vi "SYSID_FPGA2.vi"() -> ()   [LabVIEW 2014, in "SYSID.lvlib"]
doc: "This VI was generated automatically using the FPGA Wizard. You can modify the VI normally."
uses:
  SYSID.lvlib
  <vilib>/Platform/TimedLoop/XDataNode/timing_clust.ctl
  <vilib>/Platform/TimedLoop/XDataNode/nitl_modes.ctl
  <vilib>/Platform/TimedLoop/XDataNode/wakeup.ctl
  <vilib>/rvi/FXPMathLib/FxpConvert/subVIs/nifxpmath_Convert_SimConfig.ctl
  <vilib>/fxp/LVFixedPointQuantizationPolicyTypeDef.ctl
  <vilib>/fxp/LVFixedPointOverflowPolicyTypeDef.ctl
  <vilib>/rvi/Emulation/niFpgaGetClockAttributes.vi
  <vilib>/rvi/Emulation/niFpgaSctlEmulationGetInTimedLoop.vi
  <vilib>/rvi/Emulation/niFpgaEmulationReportErrorSimple.vi
  <vilib>/rvi/Emulation/niFpgaCriticalErrorInLSC.vi
  <vilib>/rvi/Emulation/niFpgaProcessEmulError.vi
  <vilib>/rvi/eio/common/nirviEmuTemplateMethod_errors.vi
  <vilib>/rvi/FXPMathLib/FxpConvert/simVIs/DllFxpConvertTemp_sub.vi
  <vilib>/Platform/TimedLoop/XDataNode/XDataNode.xnode
  <vilib>/eio/EIONode/EIONode.xnode
  <vilib>/rvi/FXPMathLib/FxpSub/XNode/nifxpmath_Sub.xnode
  <vilib>/rvi/FXPMathLib/FxpMul/XNode/nifxpmath_Multiplier.xnode
  <vilib>/rvi/FXPMathLib/FxpAdd/XNode/nifxpmath_Add.xnode
  <vilib>/rvi/FXPMathLib/FxpConvert/XNode/nifxpmath_Convert.xnode
  <vilib>/Platform/TimedLoop/XDataNode/XDNodeRunTimeDep.lvlib
  <vilib>/rvi/FXPMathLib/sim/FxpSim.dll
panel:
  in  "State_Control":fxp<+/-,20,5>
  in  "K4":fxp<+/-,32,7>
  in  "K3":fxp<+/-,32,7>
  in  "K2":fxp<+/-,32,7>
  in  "K1":fxp<+/-,32,7>
  out "Delta_theta":fxp<+/-,33,33>
  out "Delta_X":fxp<+/-,33,33>
  out "Pendulum Position":i32
  out "_Pendulum Position":i32
  in  "Pendulum Reset":bool
  out "Amp Cpmmand":fxp<+/-,20,5>
  in  "Reference":i32
  out "Right Limit":bool
  out "Left Limit":bool
  in  "Brake":bool=TRUE
  in  "Amp Reset":bool=TRUE
  in  "Amp Enable":bool
  in  "DGain":fxp<+/-,32,7>
  in  "PGain":fxp<+/-,32,7>
  out "Error-dot":fxp<+/-,55,34>
  out "Error":fxp<+/-,33,33>
  out "Control Late? (Latched)":bool
  out "Actual Control Rate (Ticks)":u32
  in  "Control Reset":bool
  in  "Control Rate (ticks)":u32=1000 caption="Control Rate (Ticks)"
  out "quad saved (Port0/DIO0,Port0/DIO1)":cluster{"Position":i32, "Index Count":u16}
  out "Stage Position":i32
  out "_quad pos (Port0/DIO0,Port0/DIO1)":i32
  in  "quad reset (Port0/DIO0,Port0/DIO1)":bool
  out "_quad saved (Port0/DIO0,Port0/DIO1)":cluster{"Position":i32, "Index Count":u16}
  in  "AO (ModB/AO2)":fxp<+/-,20,5>
  in  "Drive Command":fxp<+/-,20,5>
  out "AI (ModA/AI0)":fxp<+/-,26,5> format="%.6g"
  in  "Local Stop 0":bool
  out "Actual Loop Rate (Ticks)":u32
  out "Late? Latched":bool
  in  "Loop Rate (Ticks)":u32=571
  in  "Reset":bool
  in  "Start 0":bool
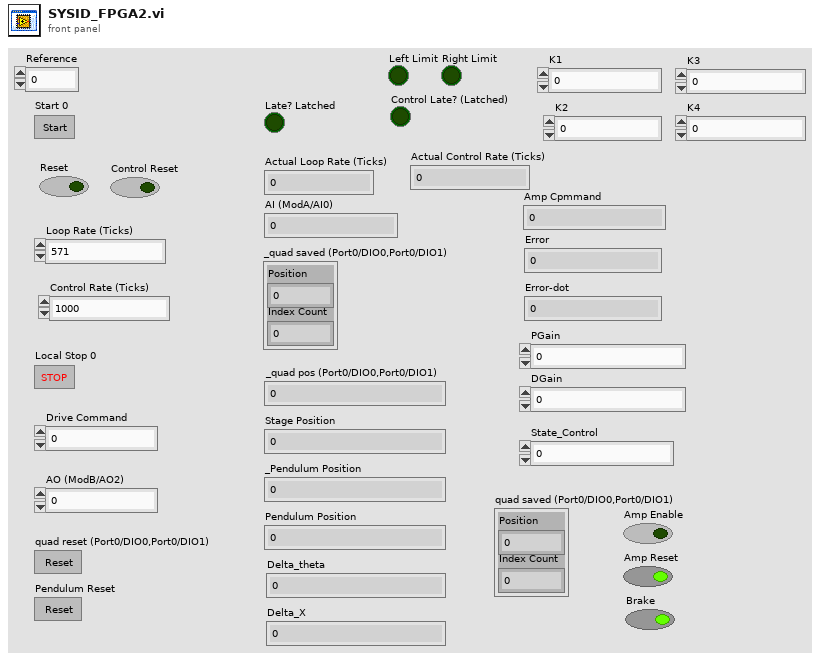
[diagram p1: front panel]
types:
  T1 = typedef "XDNodeRunTimeDep.lvlib/timing_clust.ctl" = cluster{"Expected End [f-1]":u64, "Actual End [f-1]":u64, "Finished Late? [f-1]":bool, "Expected End [i-1]":u64, "Actual End [i-1]":u64, "Finished Late? [i-1]":bool, "Expected Start [i]":u64, "Actual Start [i]":u64, "Expected Start [f]":u64, "Actual Start [f]":u64, "Source Name":string, "Structure Name":string, "Period":i64, "Deadline":i64, "Offset":i64, "Start":i64, "Priority":i32, "Timeout":i32, "Mode":T2, "Wakeup Reason":T3, "Error":errorcluster, "Source Type":string, "Secondary Source Type":string, "Global End Time":u64, "Global Start Time":u64, "Frame Duration":u64, "Iteration Duration":u64, "Assigned CPU":i32, "I/O Scan Engine Mode":u32}
  T2 = typedef "XDNodeRunTimeDep.lvlib/nitl_modes.ctl" = enum32{"No Change", "Process missed periods, maintain original phase", "Discard missed periods, maintain original phase", "Process missed periods, ignore original phase", "Discard missed periods, ignore original phase"}
  T3 = typedef "XDNodeRunTimeDep.lvlib/wakeup.ctl" = enum32{"Normal", "Aborted", "Asynchronous wakeup", "Timing source error", "Timed loop error", "Timeout"}
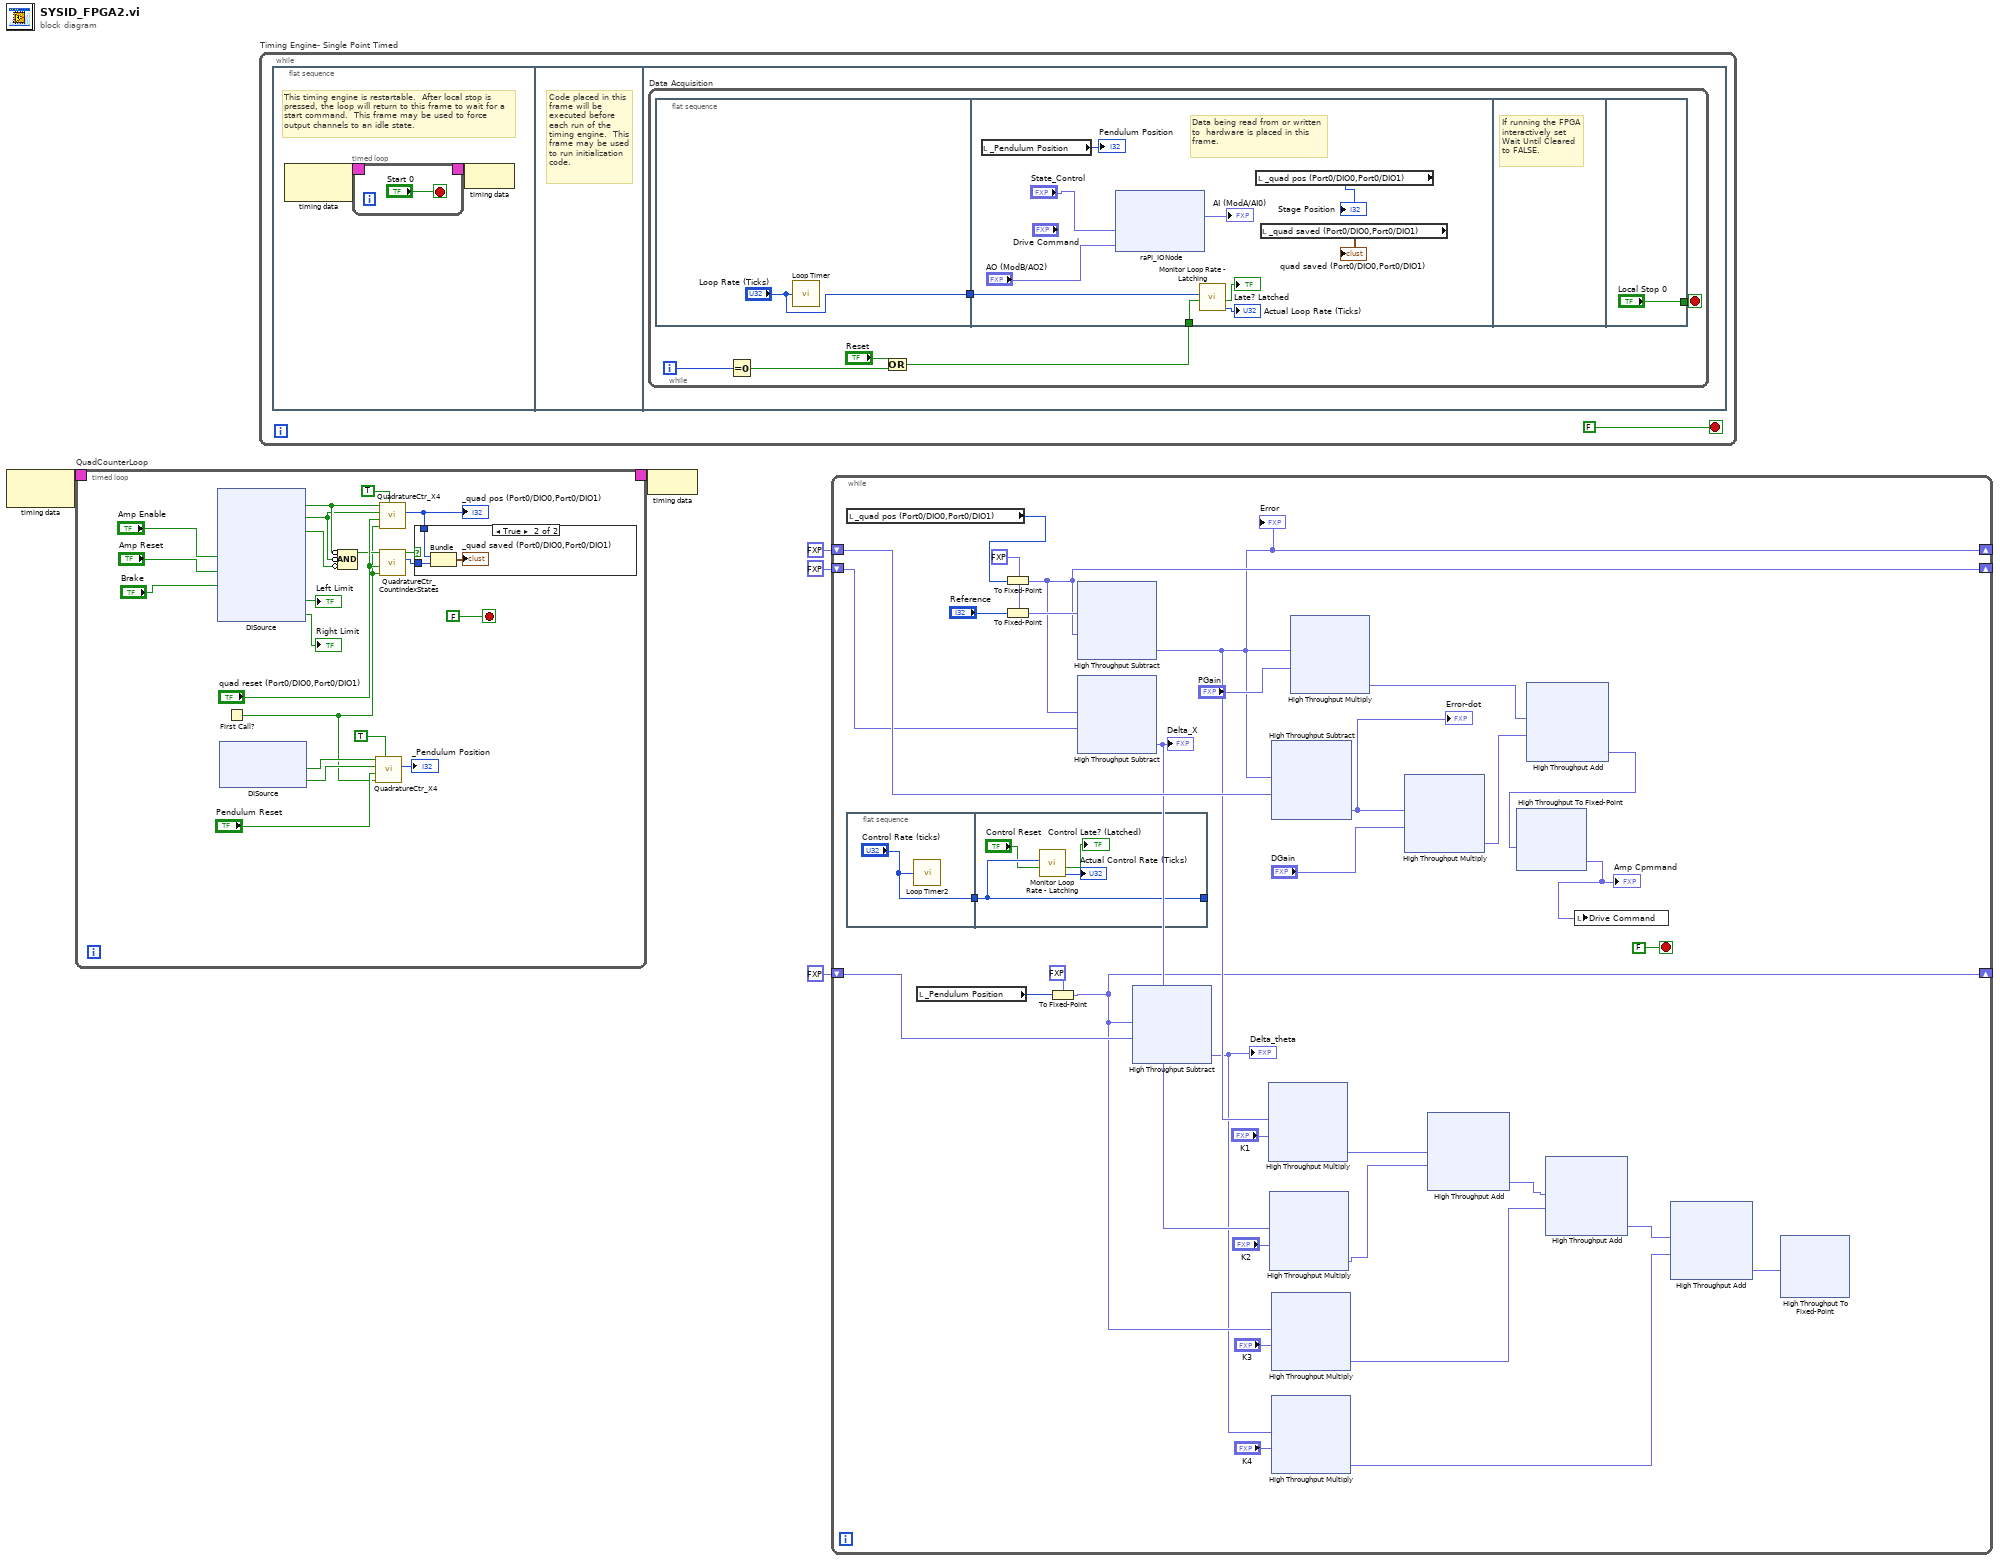
[diagram p0: block diagram]
diagram:
  n1 = node-c288 ("Input Node")() -> (w5:T1)  [unwired: 1 in]
  n2 = timed-loop "QuadCounterLoop" {
    timing: w5 -> [_]
    timing-out: [_] -> w4
    stop <- FALSE stop-if-true
    n3 = xnode ("DISource")("Port3/DIO4"="Amp Enable", "Port3/DIO8"="Amp Reset", "Port3/DIO3"="Brake") -> ("Port3/DIO0"=w20:bool, "Port3/DIO1"=w19:bool, "Port3/DIO2"=w18:bool, "Port3/DIO5"=→"Left Limit":bool, "Port3/DIO6"=→"Right Limit":bool)  [unwired: 8 in, 8 out]
    n4 = xnode ("DISource")() -> ("Port7/DIO0"=w10:bool, "Port7/DIO1"=w9:bool)  [unwired: 2 in, 2 out]
    n5 = First Call?() -> (First Call?: T/F=w7:bool)
    n6 = Compound Arithmetic op=AND(invert w20, invert w19, invert w18) -> (w17:bool)
    n7 = call "QuadratureCtr_X4.vi"("Direction?"=TRUE, "First Run?"=w7, "Reset"="Pendulum Reset", "Source B"=w9, "Source A"=w10) -> ("Position"=→"_Pendulum Position":i32)  [unwired: 6 in]
    n8 = call "QuadratureCtr_X4.vi"("Direction?"=TRUE, "First Run?"=w7, "Reset"="quad reset (Port0/DIO0,Port0/DIO1)", "Source B"=w19, "Source A"=w20) -> ("Position"=w24:i32)  [unwired: 6 in]
    "_quad pos (Port0/DIO0,Port0/DIO1)" <- w24
    n9 = call "QuadratureCtr_CountIndexStates.vi"("First Run?"=w7, "Reset"="quad reset (Port0/DIO0,Port0/DIO1)", "Valid Index State?"=w17) -> ("Index State Count"=w22:u16, "Save State?"=w21:bool)  [unwired: 7 in]
    n10 = case shown="True" w21 {
      tunnel: w24 -> [_ w29]
      tunnel: w22 -> [_ w27]
      frame False {
      }
      frame True {
        n11 = Bundle("Position"=w29, "Index State Count"=w27) -> (→"_quad saved (Port0/DIO0,Port0/DIO1)":cluster{"Position":i32, "Index State Count":u16})  [unwired: 1 in]
      }
    }
  }
  n12 = while "Timing Engine- Single Point Timed" {
    stop <- FALSE stop-if-true
    n13 = flat-sequence "MainSeq" {
      frame #0 {
        # "This timing engine is restartable.  After local stop is pressed, the loop will return to this frame to wait for a start command.  This frame may be used to force output channels to an idle state."
        n14 = node-c288 ("Input Node")() -> (w34:T1)  [unwired: 1 in]
        n15 = timed-loop "initWait" {
          timing: w34 -> [_]
          timing-out: [_] -> w33
          stop <- "Start 0" stop-if-true
        }
        n16 = node-c288 ("Output Node")(w33) -> ()
      }
      frame #1 {
        # "Code placed in this frame will be executed before each run of the timing engine.  This frame may be used to run initialization code."
      }
      frame #2 {
        n17 = while "Data Acquisition" {
          i -> [w43]
          stop <- w45 stop-if-true
          n18 = flat-sequence "Data Acquisition Sequence" {
            tunnel: ["Loop Rate (Ticks)"] -> w44
            tunnel: w44 -> [w54]
            tunnel: w40 -> [w53]
            tunnel: ["Local Stop 0"] -> w45
            frame #0 {
              n19 = call "Loop Timer"("Count(Ticks)"="Loop Rate (Ticks)") -> ()  [unwired: 1 out]
            }
            frame #1 {
              # "Data being read from or written to  hardware is placed in this frame."
              n20 = local read "_Pendulum Position"() -> (→"Pendulum Position":i32)
              n21 = xnode ("raPI_IONode")("ModB/AO0"="State_Control", "ModB/AO2"="AO (ModB/AO2)") -> ("ModA/AI0"=→"AI (ModA/AI0)":fxp<+/-,26,5>)  [unwired: 3 in, 3 out]
              n22 = call "Monitor Loop Rate - Latching.vi"("Reset"=w53, "Count(Ticks)"=w54) -> ("Actual Loop Rate (Ticks)"=→"Actual Loop Rate (Ticks)":u32, "Late? (Latched)"=→"Late? Latched":bool)  [unwired: 7 in, 1 out]
              n23 = local read "_quad pos (Port0/DIO0,Port0/DIO1)"() -> (→"Stage Position":i32)
              n24 = local read "_quad saved (Port0/DIO0,Port0/DIO1)"() -> (→"quad saved (Port0/DIO0,Port0/DIO1)":cluster{"Position":i32, "Index Count":u16})
            }
            frame #2 {
              # "If running the FPGA interactively set Wait Until Cleared to FALSE."
            }
            frame #3 {
            }
          }
          n25 = Equal To 0?(x=w43) -> (x = 0?=w42:bool)
          n26 = Or(x="Reset", y=w42) -> (x .or. y?=w40:bool)
        }
      }
    }
  }
  n27 = node-c288 ("Output Node")(w4) -> ()
  n28 = while {
    shift-right: [w72] -> _
    shift-left: fxp<+/-,54,33> 0.0 ("x-y") -> [w90]
    shift-right: [w76] -> _
    shift-left: fxp<+/-,32,32> 0.0 ("y") -> [w77]
    shift-right: [w70] -> _
    shift-left: fxp<+/-,32,16> 0.0 ("fixed-point type") -> [w75]
    stop <- FALSE stop-if-true
    w79 = fxp<+/-,32,32> 0.0 ("y")
    n29 = local read "_quad pos (Port0/DIO0,Port0/DIO1)"() -> (w91:i32)
    n30 = flat-sequence {
      tunnel: ["Control Rate (ticks)"] -> w87
      tunnel: [w118] -> _
      tunnel: w87 -> [w118]
      frame #0 {
        n31 = call "Loop Timer2"("Count(Ticks)"="Control Rate (ticks)") -> ()  [unwired: 1 out]
      }
      frame #1 {
        n32 = call "Monitor Loop Rate - Latching.vi"("Reset"="Control Reset", "Count(Ticks)"=w118) -> ("Actual Loop Rate (Ticks)"=→"Actual Control Rate (Ticks)":u32, "Late? (Latched)"=→"Control Late? (Latched)":bool)  [unwired: 7 in, 1 out]
      }
    }
    n33 = local read "_Pendulum Position"() -> (w73:i32)
    n34 = To Fixed-Point(fixed-point type=w79, number=w91) -> (fixed-point=w76:fxp<+/-,32,32>)
    n35 = To Fixed-Point(fixed-point type=w79, number="Reference") -> (fixed-point=w78:fxp<+/-,32,32>)
    n36 = To Fixed-Point(fixed-point type=fxp<+/-,32,16> 0.0, number=w73) -> (fixed-point=w70:fxp<+/-,32,16>)
    n37 = xnode "High Throughput Subtract"("x"=w78, "y"=w76) -> ("x-y"=w72:fxp<+/-,33,33>)
    "Error" <- w72
    n38 = xnode "High Throughput Subtract"("x"=w76, "y"=w77) -> ("x-y"=w71:fxp<+/-,33,33>)
    "Delta_X" <- w71
    n39 = xnode "High Throughput Subtract"("x"=w70, "y"=w75) -> ("x-y"=w69:fxp<+/-,33,33>)
    "Delta_theta" <- w69
    n40 = xnode "High Throughput Multiply"("x"=w72, "y"="K1") -> ("x*y"=w64:fxp<+/-,64,40>)
    n41 = xnode "High Throughput Multiply"("x"=w71, "y"="K2") -> ("x*y"=w63:fxp<+/-,64,40>)
    n42 = xnode "High Throughput Multiply"("x"=w70, "y"="K3") -> ("x*y"=w61:fxp<+/-,64,23>)
    n43 = xnode "High Throughput Multiply"("x"=w69, "y"="K4") -> ("x*y"=w59:fxp<+/-,64,40>)
    n44 = xnode "High Throughput Subtract"("x"=w72, "y"=w90) -> ("x-y"=w89:fxp<+/-,55,34>)
    "Error-dot" <- w89
    n45 = xnode "High Throughput Multiply"("x"=w72, "y"="PGain") -> ("x*y"=w85:fxp<+/-,64,40>)
    n46 = xnode "High Throughput Multiply"("x"=w89, "y"="DGain") -> ("x*y"=w84:fxp<+/-,64,41>)
    n47 = xnode "High Throughput Add"("x"=w64, "y"=w63) -> ("x+y"=w62:fxp<+/-,64,41>)
    n48 = xnode "High Throughput Add"("x"=w85, "y"=w84) -> ("x+y"=w83:fxp<+/-,64,42>)
    n49 = xnode "High Throughput To Fixed-Point"("x"=w83) -> ("y"=w88:fxp<+/-,20,5>)
    "Amp Cpmmand" <- w88
    n50 = xnode "High Throughput Add"("x"=w62, "y"=w61) -> ("x+y"=w60:fxp<+/-,64,42>)
    n51 = local write "Drive Command"(w88) -> ()
    n52 = xnode "High Throughput Add"("x"=w60, "y"=w59) -> ("x+y"=w58:fxp<+/-,64,43>)
    n53 = xnode "High Throughput To Fixed-Point"("x"=w58) -> ()  [unwired: 1 out]
  }
